vi "IT6700H Step Make.vi"() -> ()   [LabVIEW 2015]
uses:
  <instrlib>/IT6700H/IT6700H.lvlib
panel:
  in  "Step Value":dbl=0.5 format="%.2f"
  in  "Function":u16(ring) items=["Voltage", "Current"]
  in  "Step Type":u16(ring) items=["Up", "Down"]
  in  "Serial Configuration":T1={"Baud Rate"=9600, "Parity"=0, "Data Bits"=8, "Stop Bits"=10, "Flow Control"=0} {"Flow Control" items=["None", "XON/XOFF", "RTS/CTS", "XON/XOFF & RTS/CTS", "DTR/DSR", "XON/XOFF & DTR/DSR"]; "Stop Bits" items=["1.0"=10, "1.5"=15, "2.0"=20]; "Data Bits" items=["7"=7, "8"=8]; "Parity" items=["None", "Odd", "Even", "Mark", "Space"]; "Baud Rate" items=["300"=300, "600"=600, "1200"=1200, "2400"=2400, "4800"=4800, "9600"=9600, "19200"=19200]}
  in  "Stop Output":bool
  in  "Initial Level":dbl format="%.2f"
  out "Actual Level":dbl format="%.3f"
  in  "End Level":dbl=10.0 format="%.2f"
  in  "VISA resource name":refnum<visa-resource-name>
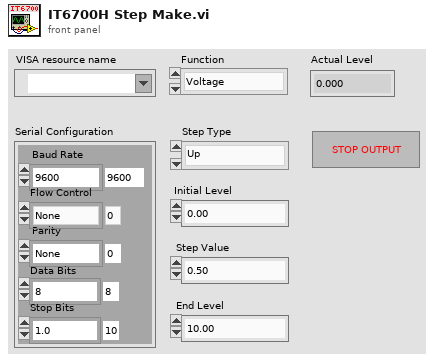
[diagram p1: front panel]
types:
  T1 = cluster{"Baud Rate":u32, "Parity":u16, "Data Bits":u16, "Stop Bits":u16, "Flow Control":u16}
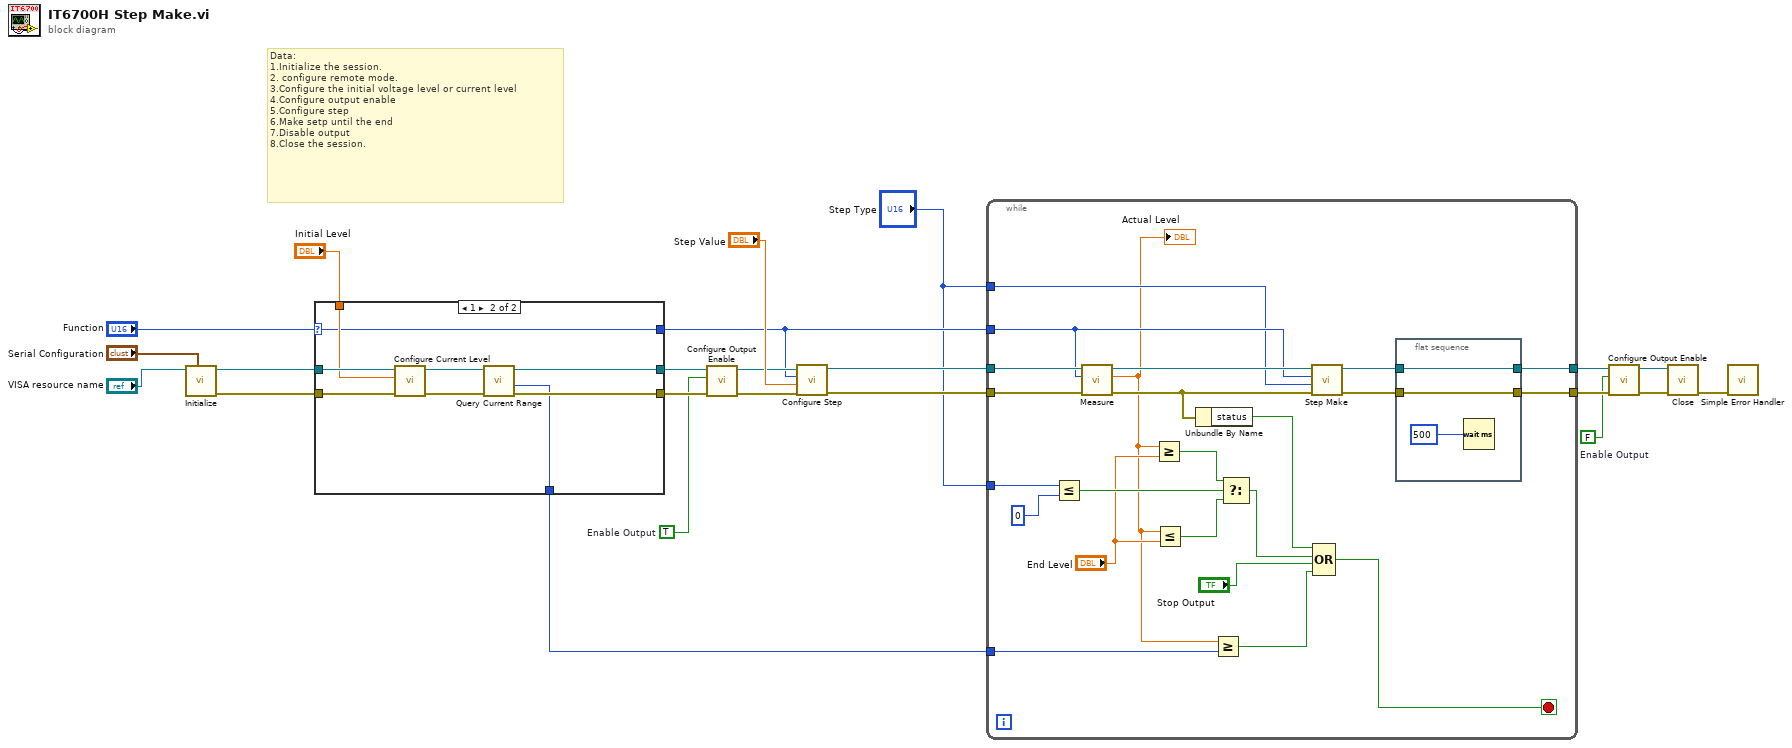
[diagram p0: block diagram]
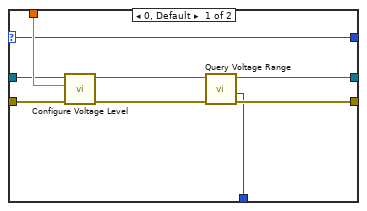
[diagram p2: hidden frame]
diagram:
  w7 = FALSE  # Enable Output
  w17 = TRUE  # Enable Output
  # "Data:\n1.Initialize the session.\n2. configure remote mode.\n3.Configure the initial voltage level or current level\n4.Configure output enable\n5.Configure step\n6.Make setp until the end\n7.Disable output\n8.Close the session."
  n1 = call <instrlib>:"Initialize.vi"("Serial Configuration"="Serial Configuration", "VISA resource name"="VISA resource name") -> ("error out"=w2:errorcluster, "VISA resource name out"=w3:refnum<visa-resource-name>)  [unwired: 8 in]
  n2 = case "条件结构" shown="1" "Function" {
    selector: "Function" -> [w29 w38]
    tunnel: "Initial Level" -> [w32 w39]
    tunnel: w3 -> [w31 w41]
    tunnel: w2 -> [w30 w40]
    tunnel: [w26 w34] -> w19
    tunnel: [w25 w35] -> w18
    tunnel: [w29 w38] -> w11
    tunnel: [w24 w33] -> w1
    frame 0, Default {
      n3 = call <instrlib>:"Configure Voltage Level.vi"("error in (no error)"=w30, "Voltage Level (0.0 V)"=w32, "VISA resource name"=w31) -> ("error out"=w27:errorcluster, "VISA resource name out"=w28:refnum<visa-resource-name>)  [unwired: 7 in]
      n4 = call <instrlib>:"Query Voltage Range.vi"("error in (no error)"=w27, "VISA resource name"=w28) -> ("error out"=w25:errorcluster, "Maximum value"=w24:u16, "VISA resource name out"=w26:refnum<visa-resource-name>)  [unwired: 6 in, 1 out]
    }
    frame 1 {
      n5 = call <instrlib>:"Configure Current Level.vi"("error in (no error)"=w40, "Current Level (0.0 A)"=w39, "VISA resource name"=w41) -> ("error out"=w36:errorcluster, "VISA resource name out"=w37:refnum<visa-resource-name>)  [unwired: 7 in]
      n6 = call <instrlib>:"Query Current Range.vi"("error in (no error)"=w36, "VISA resource name"=w37) -> ("error out"=w35:errorcluster, "Maximum value"=w33:u16, "VISA resource name out"=w34:refnum<visa-resource-name>)  [unwired: 6 in, 1 out]
    }
  }
  n7 = call <instrlib>:"Configure Output Enable.vi"("VISA resource name"=w19, "Enable Output (T: Enable)"=w17, "error in (no error)"=w18) -> ("VISA resource name out"=w14:refnum<visa-resource-name>, "error out"=w16:errorcluster)  [unwired: 6 in]
  n8 = call <instrlib>:"Configure Step.vi"("error in (no error)"=w16, "Step value"="Step Value", "Function"=w11, "VISA resource name"=w14) -> ("error out"=w12:errorcluster, "VISA resource name out"=w13:refnum<visa-resource-name>)  [unwired: 6 in]
  n9 = while {
    tunnel: w13 -> [w64]
    tunnel: w12 -> [w63]
    tunnel: w11 -> [w50]
    tunnel: "Step Type" -> [w62]
    tunnel: "Step Type" -> [w49]
    tunnel: [w47] -> w9
    tunnel: [w46] -> w8
    tunnel: w1 -> [w44]
    stop <- w51 stop-if-true
    n10 = Less Or Equal?(x=w62, y=0) -> (x <= y?=w60:bool)
    n11 = call <instrlib>:"Measure.vi"("error in (no error)"=w63, "Measure Type"=w50, "VISA resource name"=w64) -> ("error out"=w55:errorcluster, "Measurement"=w43:dbl, "VISA resource name out"=w56:refnum<visa-resource-name>)  [unwired: 6 in]
    "Actual Level" <- w43
    n12 = Greater Or Equal?(x=w43, y="End Level") -> (x >= y?=w58:bool)
    n13 = Less Or Equal?(x=w43, y="End Level") -> (x <= y?=w57:bool)
    n14 = Unbundle By Name(w55) -> ("status"=w54:bool)
    n15 = Greater Or Equal?(x=w43, y=w44) -> (x >= y?=w42:bool)
    n16 = Select(t=w58, s=w60, f=w57) -> (s? t:f=w53:bool)
    n17 = call <instrlib>:"Step Make.vi"("error in (no error)"=w55, "Step Type (0: UP)"=w49, "Function (0: Voltage)"=w50, "VISA resource name"=w56) -> ("error out"=w45:errorcluster, "VISA resource name out"=w48:refnum<visa-resource-name>)  [unwired: 6 in]
    n18 = Compound Arithmetic op=OR(w54, w53, "Stop Output", w42) -> (w51:bool)
    n19 = flat-sequence {
      tunnel: w48 -> [w67]
      tunnel: [w67] -> w47
      tunnel: [w66] -> w46
      tunnel: w45 -> [w66]
      frame #0 {
        n20 = Wait (ms)(milliseconds to wait=500) -> ()  [unwired: 1 out]
      }
    }
  }
  n21 = call <instrlib>:"Configure Output Enable.vi"("VISA resource name"=w9, "Enable Output (T: Enable)"=w7, "error in (no error)"=w8) -> ("VISA resource name out"=w5:refnum<visa-resource-name>, "error out"=w6:errorcluster)  [unwired: 6 in]
  n22 = call <instrlib>:"Close.vi"("error in (no error)"=w6, "VISA resource name"=w5) -> ("error out"=w4:errorcluster)  [unwired: 9 in]
  n23 = call <vilib>:"Simple Error Handler.vi"("error in (no error)"=w4) -> ()  [unwired: 4 in, 5 out]
